vi "udp send to LA.vi"() -> ()   [LabVIEW 2017]
uses:
  global variable.vi
panel:
  out "fffff":string
  in  "Stop":bool
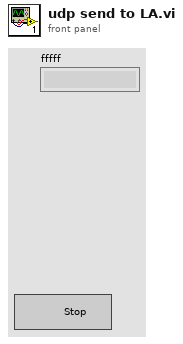
[diagram p1: front panel]
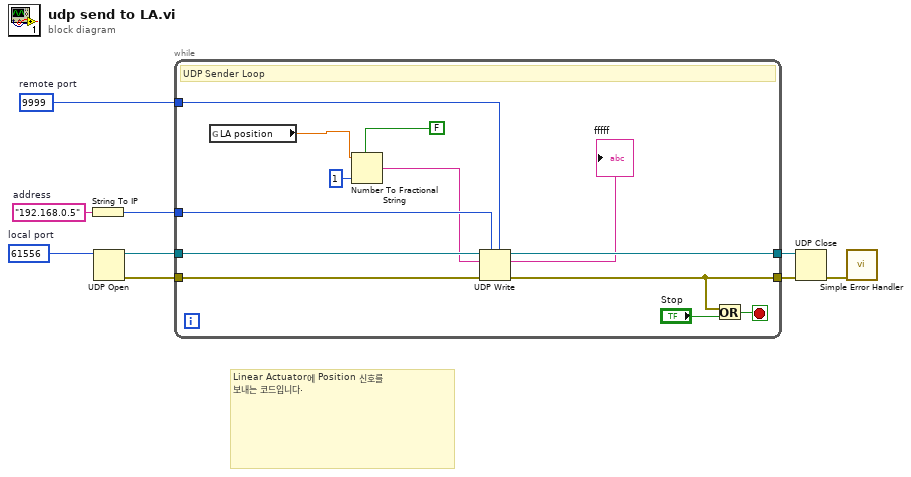
[diagram p0: block diagram]
diagram:
  w1 = u16 9999  # remote port
  w2 = u16 61556  # local port
  w7 = "192.168.0.5"  # address
  # "Linear Actuator에 Position 신호를\n보내는 코드입니다."
  n1 = String To IP(1:w7) -> (0:w5:u32)
  n2 = UDP Open(11:w2) -> (port=w4:refnum<k16>, 0:w3:errorcluster)  [unwired: 4 in, 1 out]
  n3 = while {
    tunnel: [w16] -> w8
    tunnel: w4 -> [w21]
    tunnel: w3 -> [w20]
    tunnel: [w17] -> w9
    tunnel: w5 -> [w15]
    tunnel: w1 -> [w13]
    stop <- w19 stop-if-true
    # "UDP Sender Loop"
    n4 = global read "global variable.vi" "LA position"() -> (w10:dbl)
    n5 = Number To Fractional String(use system decimal point (T)=FALSE, number=w10, precision (6)=i16 1 ("정밀도(6)")) -> (F-format string=w14:string)  [unwired: 1 in]
    "fffff" <- w14
    n6 = UDP Write(address=w15, port or service name=w13, connection ID=w21, data in=w14, 8:w20) -> (error out=w16:errorcluster, 3:w17:refnum<k16>)  [unwired: 1 in]
    n7 = Or(x=w16, y="Stop") -> (x .or. y?=w19:bool)
  }
  n8 = UDP Close(connection ID=w9, 8:w8) -> (error out=w6:errorcluster)  [unwired: 1 out]
  n9 = call <vilib>:"Simple Error Handler.vi"("error in (no error)"=w6) -> ()  [unwired: 4 in, 5 out]
